vi "FGV_REF_EDITOR_records_display.vi"(4 "front_panel_reference":refnum<vi>, 6 "SQL_listbox_reference":refnum<vi>, 7 "options":T3, 8 "error_in":errorcluster, 10 "uneditable_columns":string[](array[string])=["ID", "CREATION_TIME", "CREATED_BY"], 11 "input":variant) -> (0 "error_out":errorcluster, 1 "all_info":T1, 2 "array_param_output":string[](array[string]), 3 "string_param_output":string)   [LabVIEW 2019]
uses:
  FGV_REF_EDITOR_records_display.ctl
  REF_EDITOR_all_info.ctl
  MAIN/SQL_record_states.ctl
  ini/typedef/CLIENT_all_config_info.ctl
  ini/typedef/CLIENT_main_ini_file.ctl
  queues/typedef/CLIENT_queue_refnums.ctl
  queues/typedef/SQL_EDITOR_queue_element.ctl
  MAIN/SQL_EDITOR/SQL_EDITOR_sequence_state.ctl
  queues/typedef/CLIENT_SCANNER_queue_element.ctl
  MAIN/SCANNER/SCANNER_sequence_state.ctl
  queues/typedef/CLIENT_REF_CHG_queue_element.ctl
  MAIN/reference_changed_connection/CLIENT_REF_CHG_sequence_state.ctl
  login/FGV_login.ctl
  <userlib>/_OpenG.lib/array/array.llb/Filter 1D Array (String)__ogtk.vi
  <userlib>/_OpenG.lib/array/array.llb/Delete Elements from 1D Array (I32)__ogtk.vi
  <vilib>/addons/database/_DB Variant To Data/Database Variant To Data.xnode
panel:
  out "data":string[][](array[string])
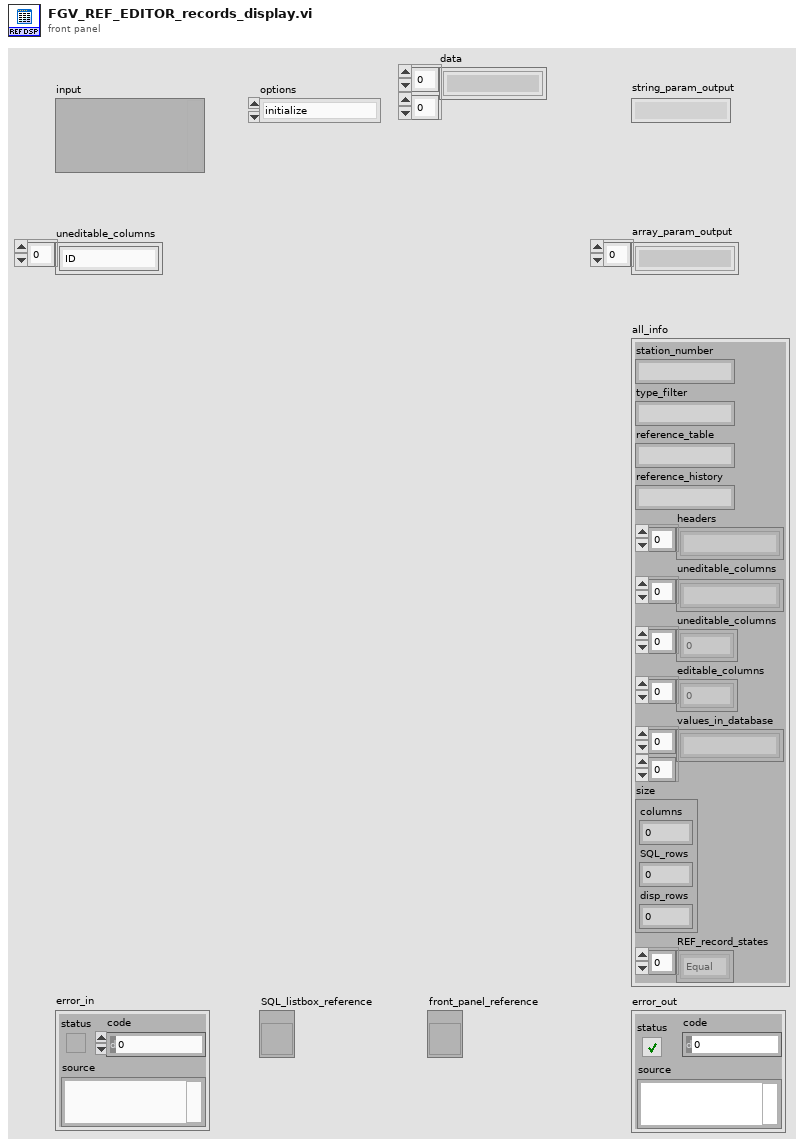
[diagram p1: front panel]
types:
  T1 = typedef "REF_EDITOR_all_info.ctl" = cluster{"station_number":string, "type_filter":string, "reference_table":string, "reference_history":string, "headers":string[], "uneditable_columns":string[], "uneditable_columns":i32[], "editable_columns":i32[], "values_in_database":string[][], "size":cluster{"columns":i32, "SQL_rows":i32, "disp_rows":i32}, "REF_record_states":T2[]}
  T2 = typedef "SQL_record_states.ctl" = enum16{"Equal", "Added", "Edited", "Deleted"}
  T3 = typedef "FGV_REF_EDITOR_records_display.ctl" = enum16{"initialize", "set_reference_tables_names", "set_station_number", "set_type_filter", "set_headers", "set_records", "get_ref_table_name", "get_ref_hist_table_name", "get_station_number", "get_type_filter", "get_headers", "get_uneditable_columns", "get_all_info", "record_added?", "record_inserted?", "record_edited?", "record_updated?", "record_deleted?", "discard_changes"}
  T4 = typedef "CLIENT_all_config_info.ctl" = cluster{"main_ini_file":T5, "SQL Password":string, "queue_refnums":T6}
  T5 = typedef "CLIENT_main_ini_file.ctl" = cluster{"SQL Driver":string, "SQL Server":string, "SQL Database":string, "SQL UID":string, "Reference table":string, "Reference history":string, "Archivisation CFG table":string, "Archivisation CFG history":string, "User table":string, "User history":string, "logout timeout [ms]":i32, "records per page":i32, "default language":string, "REF CHG connection IP":string, "REF CHG remote port":i32, "REF CHG local port":i32, "SCANNER COM port":u16, "SCANNER Baud rate":u32, "SCANNER Data bits":u16, "SCANNER Pairity":enum16{"None", "Odd", "Even", "Mark", "Space"}, "SCANNER Stop bits":u16, "SCANNER Flow control":u16, "SCANNER Termination char":u8}
  T6 = typedef "CLIENT_queue_refnums.ctl" = cluster{"SQL_EDITOR_queue":refnum<queue>, "SCANNER_queue":refnum<queue>, "SCANNER_data":refnum<queue>, "CLIENT_REF_CHG_queue":refnum<queue>}
  T7 = typedef "FGV_login.ctl" = enum16{"initialize", "login", "logout", "get_login_info"}
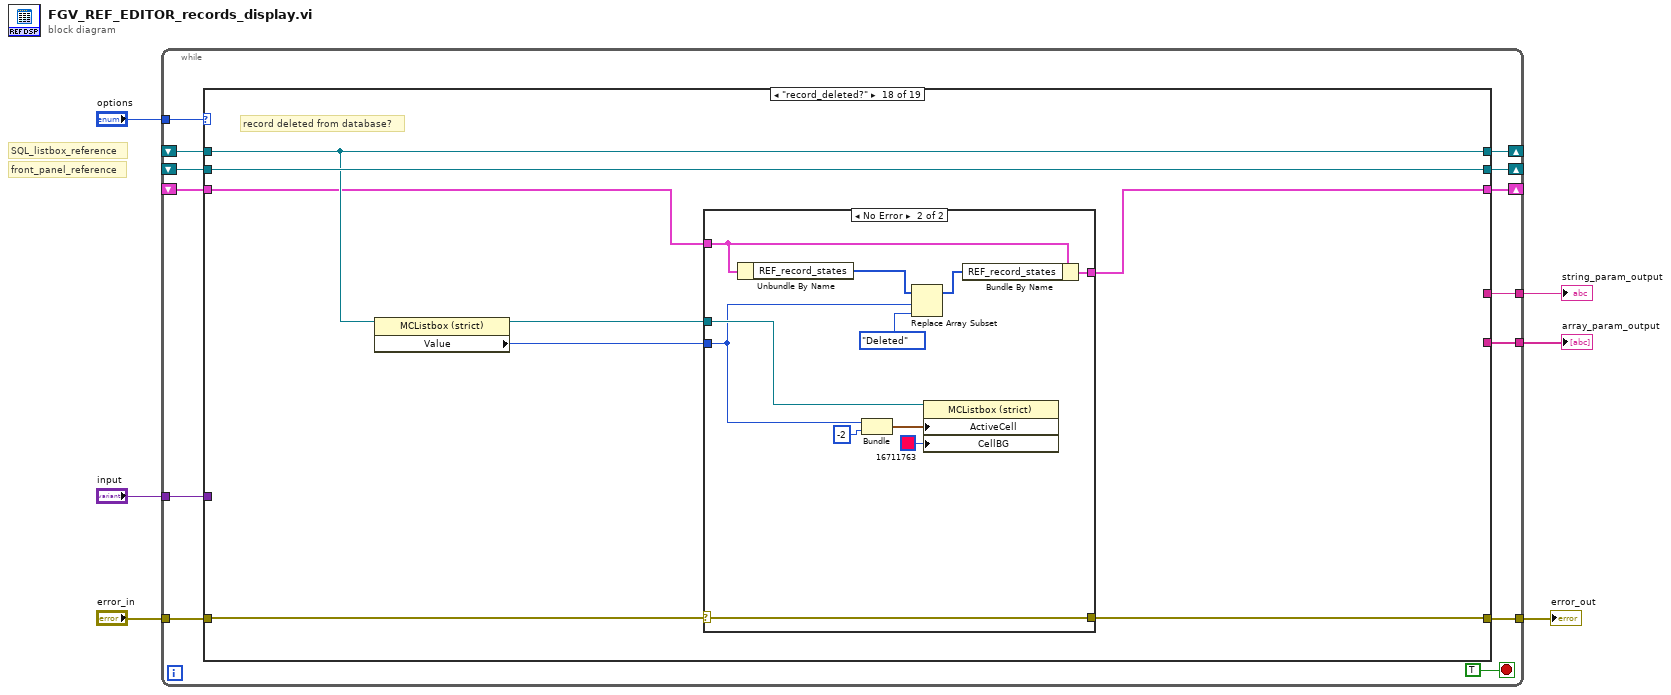
[diagram p0: block diagram]
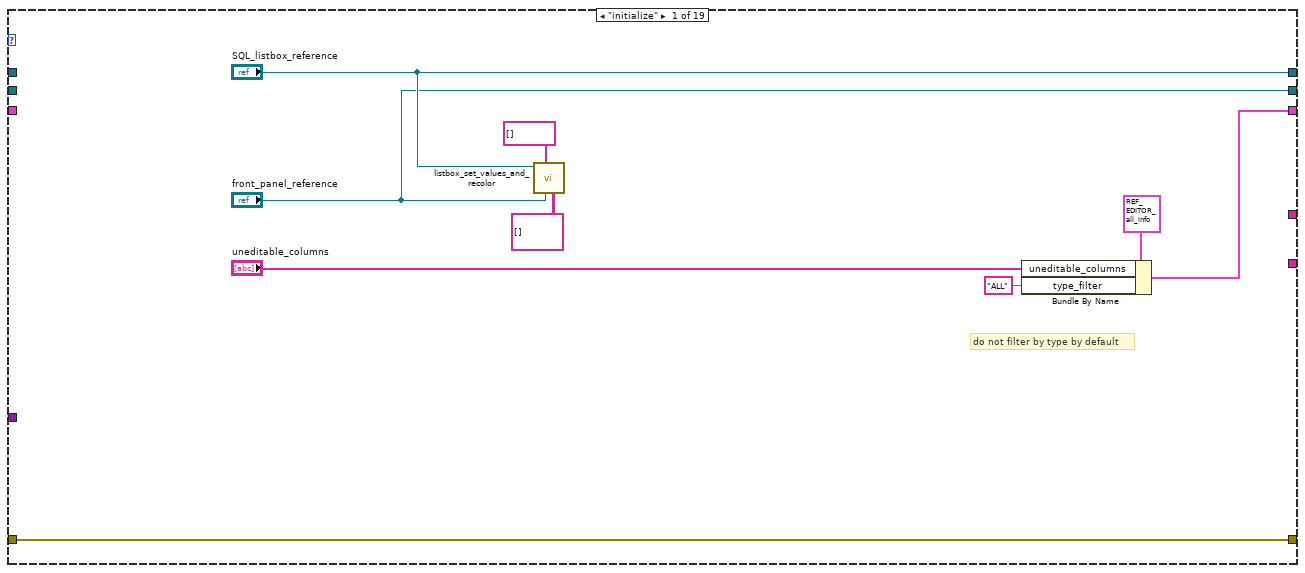
[diagram p2: hidden frame]
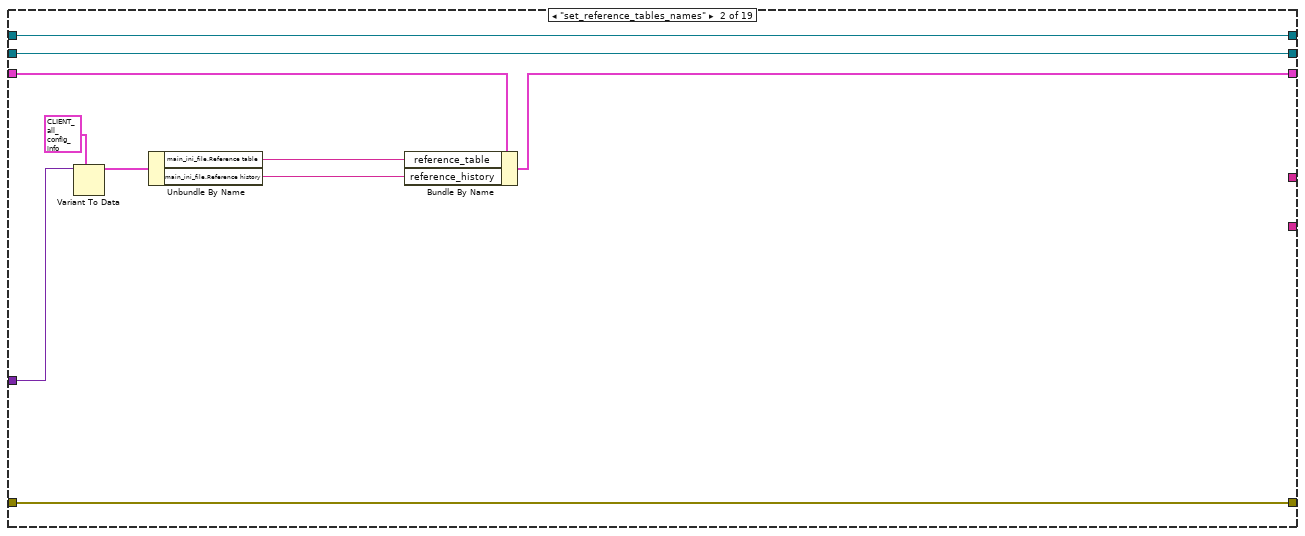
[diagram p3: hidden frame]
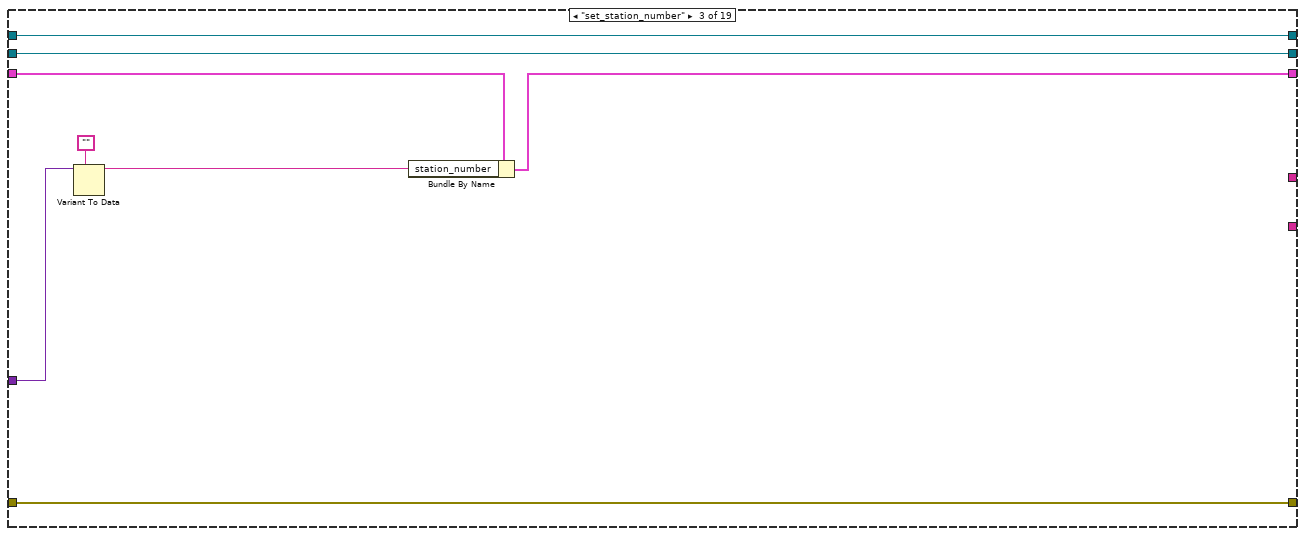
[diagram p4: hidden frame]
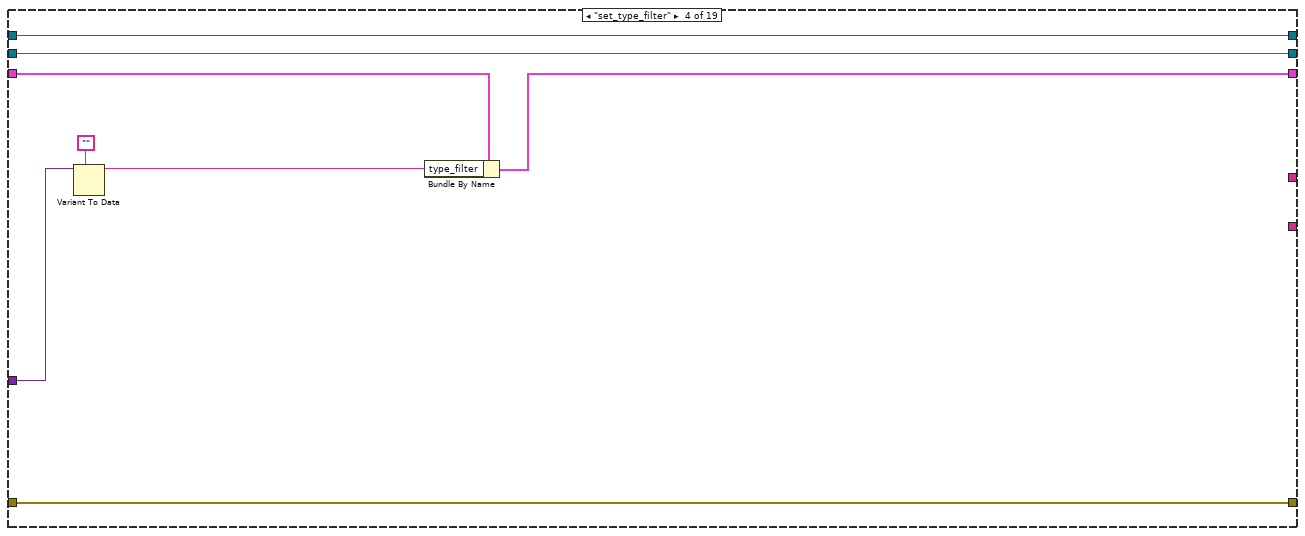
[diagram p5: hidden frame]
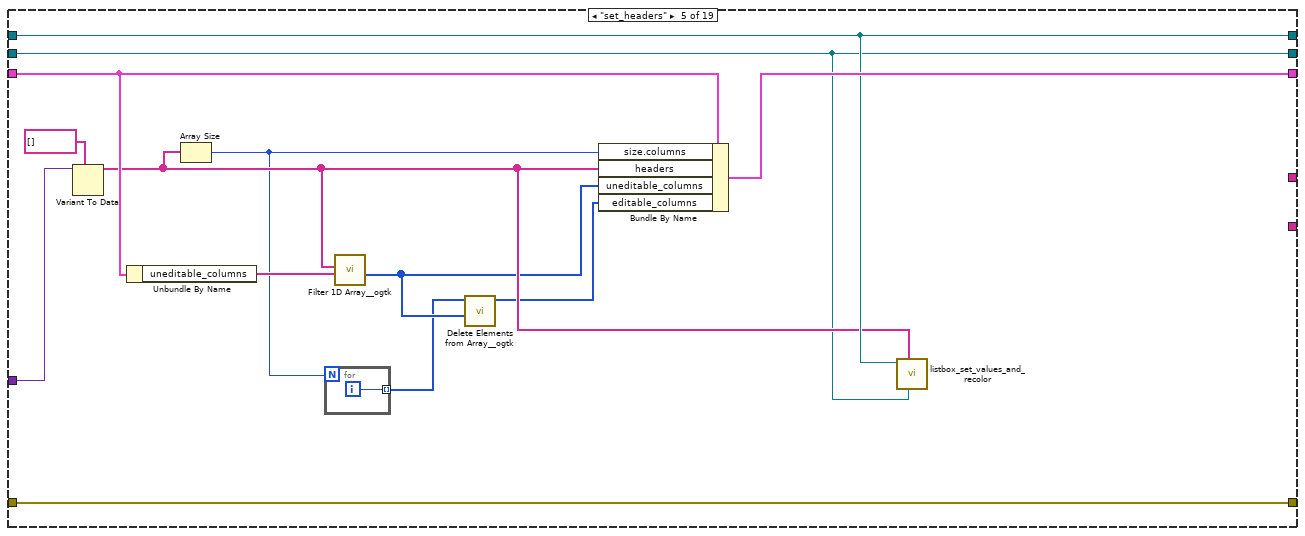
[diagram p6: hidden frame]
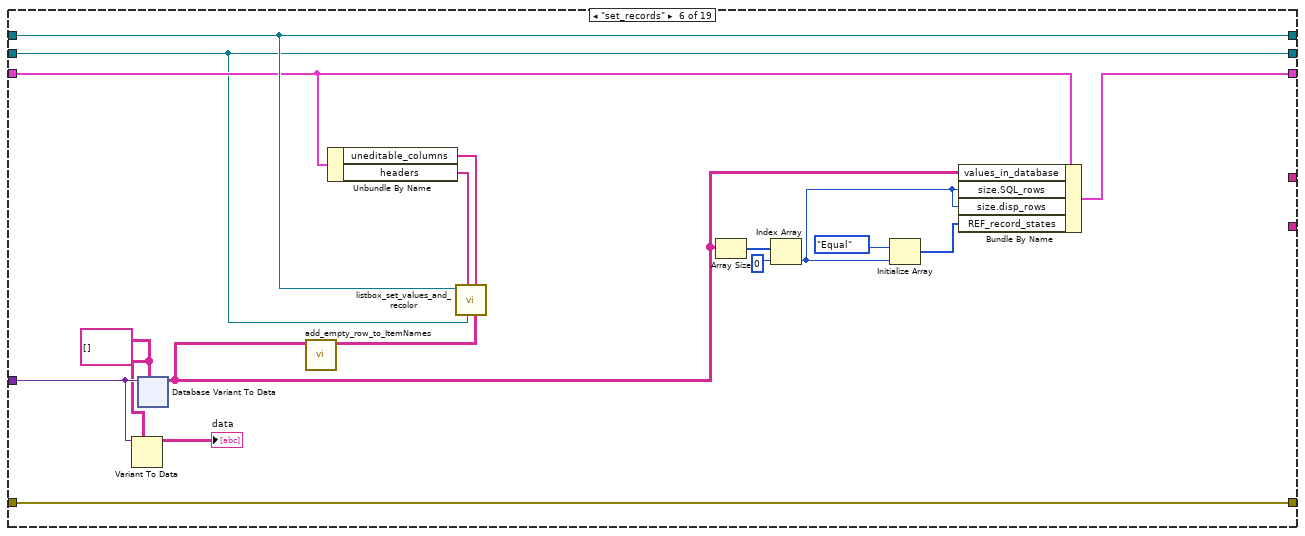
[diagram p7: hidden frame]
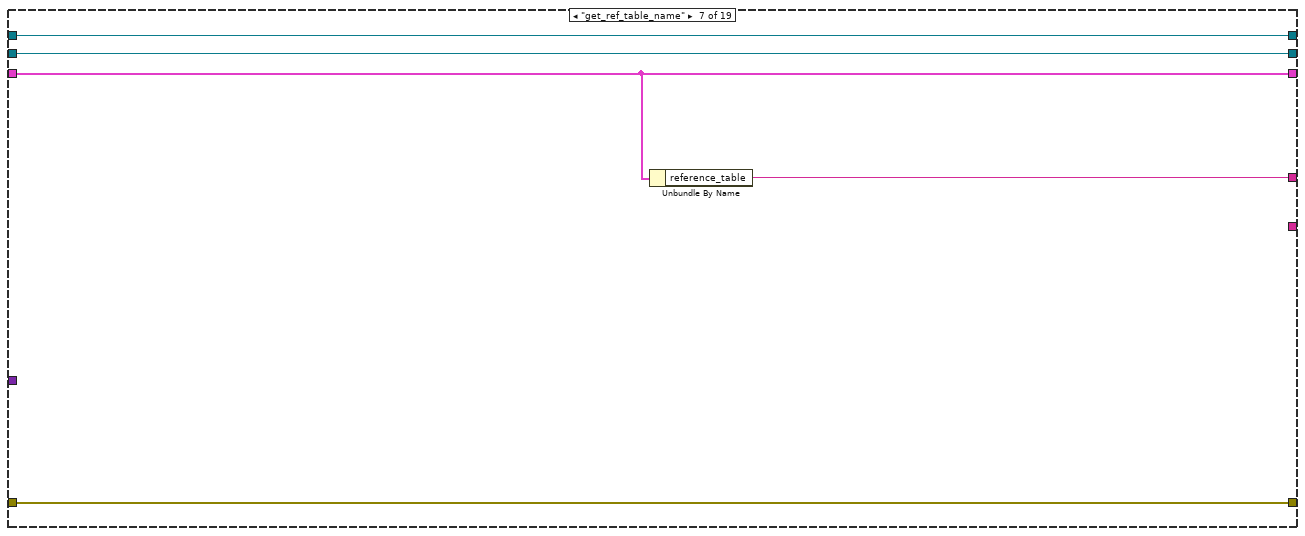
[diagram p8: hidden frame]
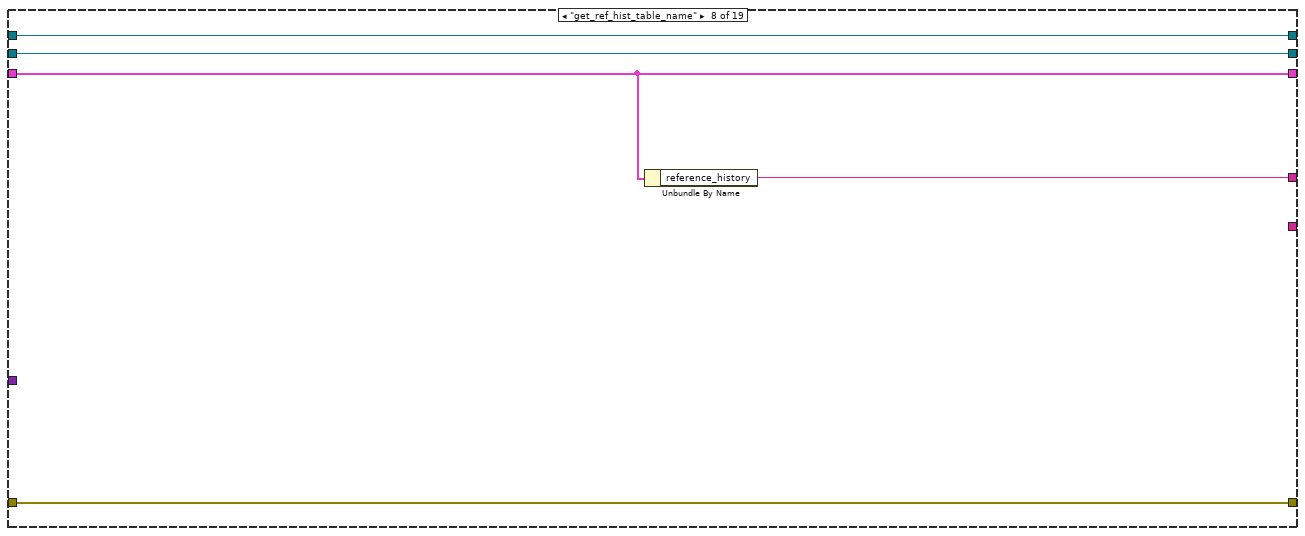
[diagram p9: hidden frame]
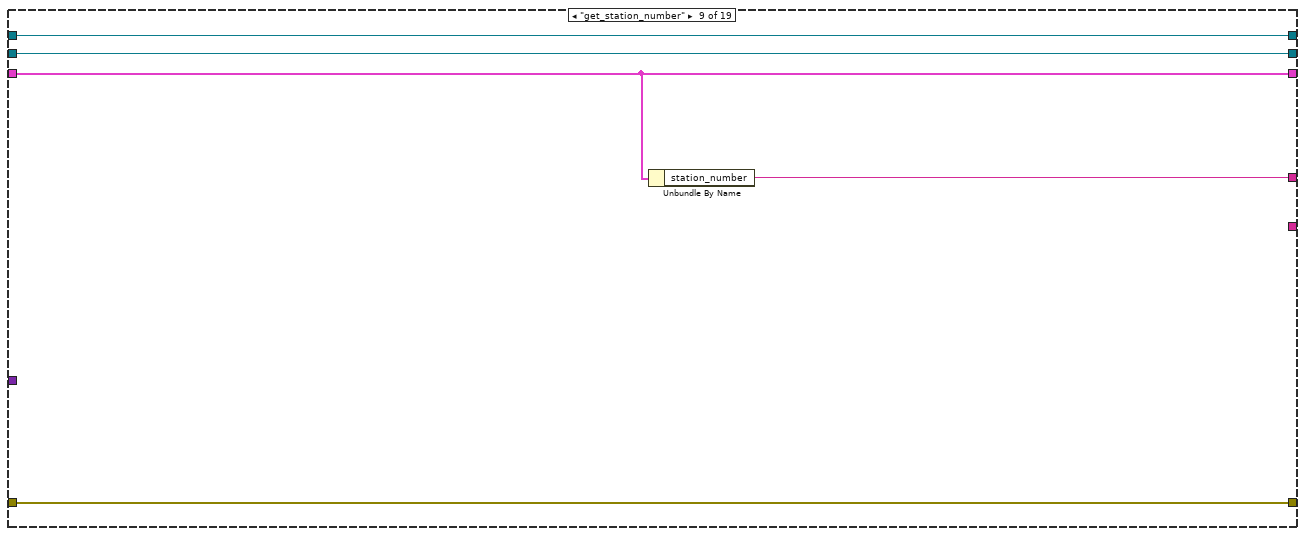
[diagram p10: hidden frame]
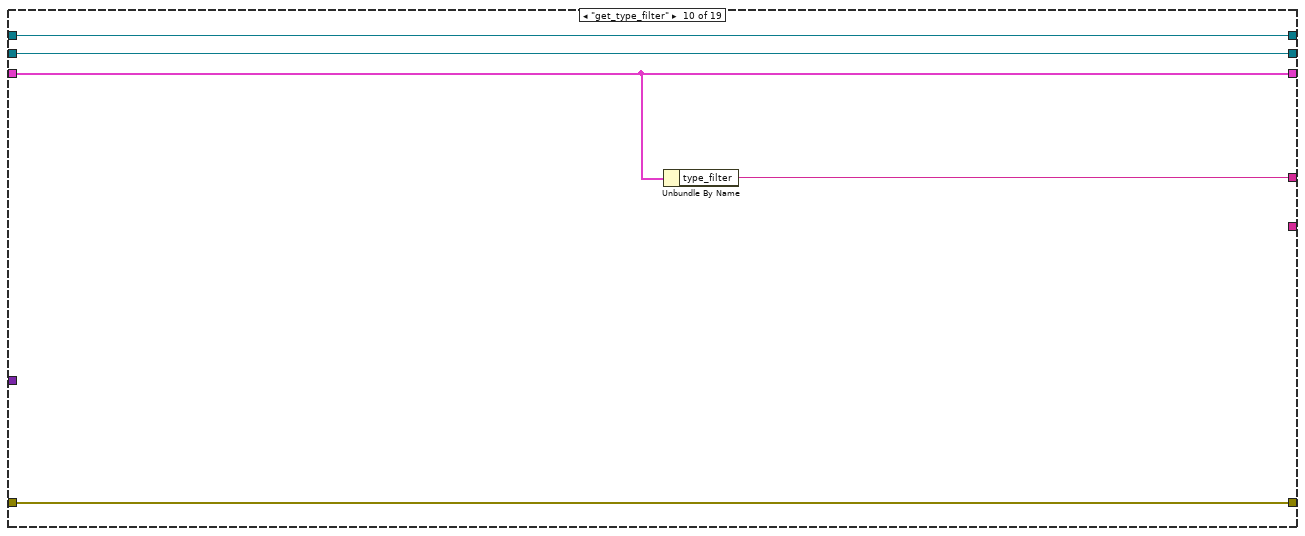
[diagram p11: hidden frame]
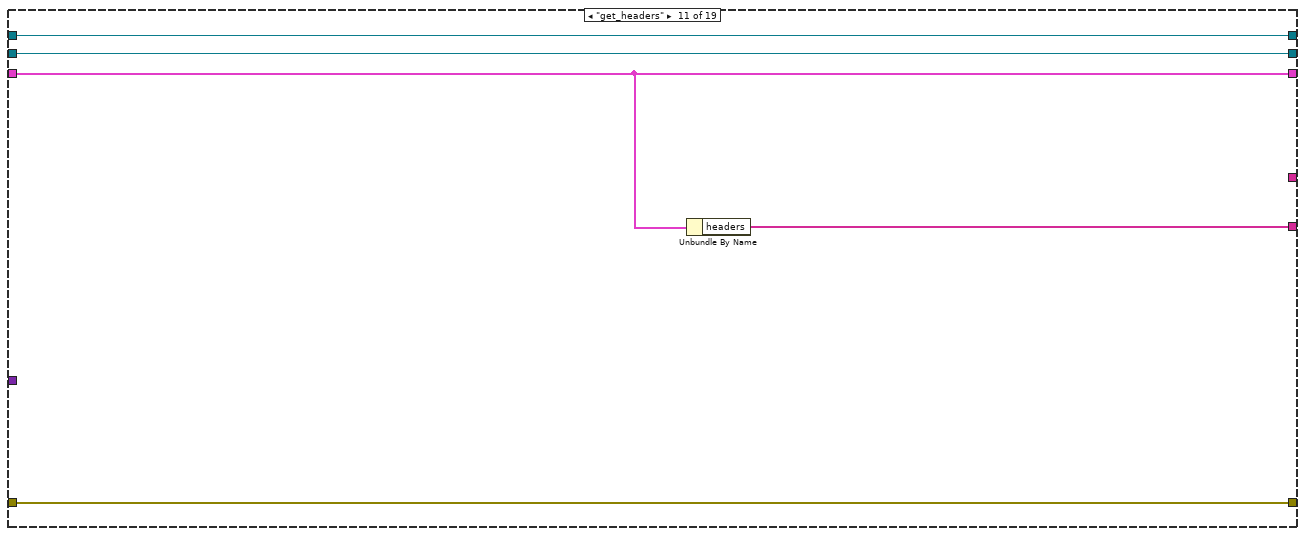
[diagram p12: hidden frame]
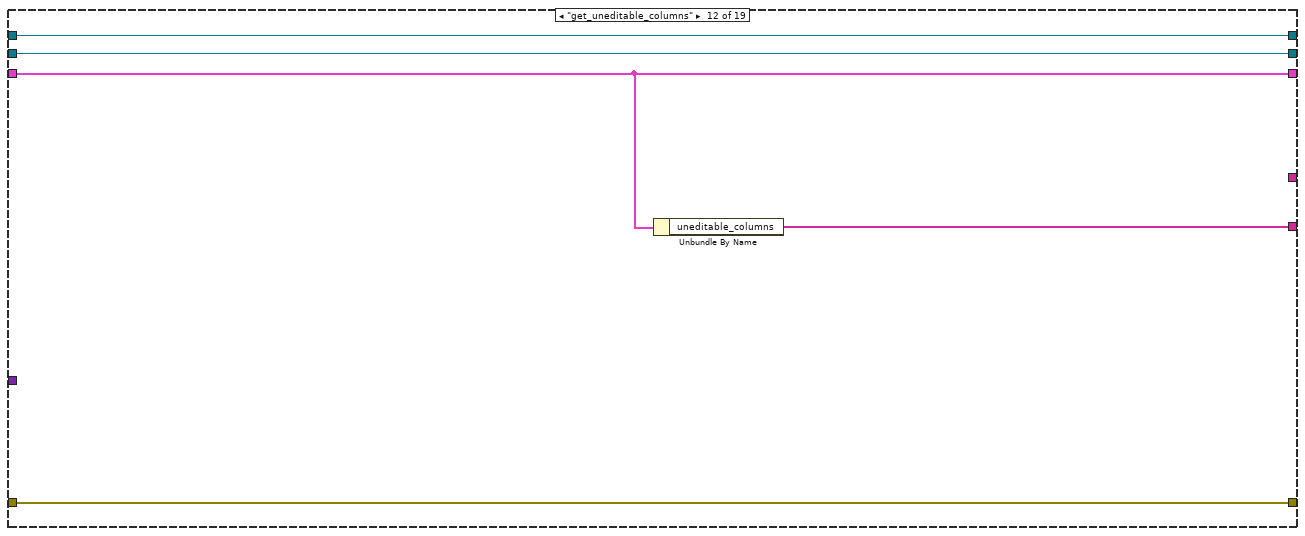
[diagram p13: hidden frame]
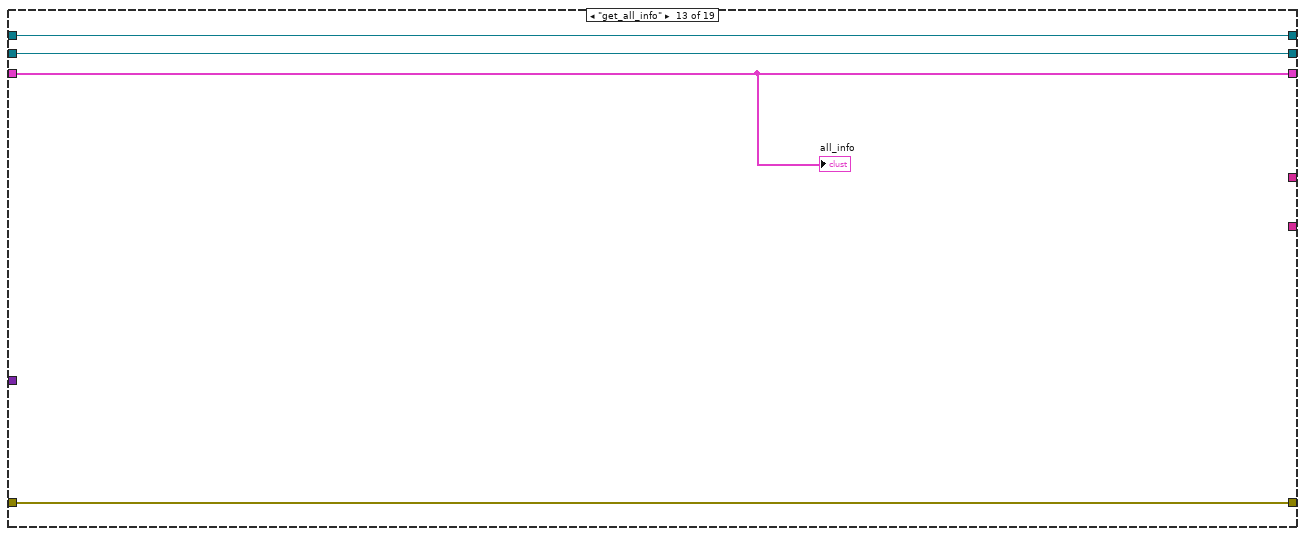
[diagram p14: hidden frame]
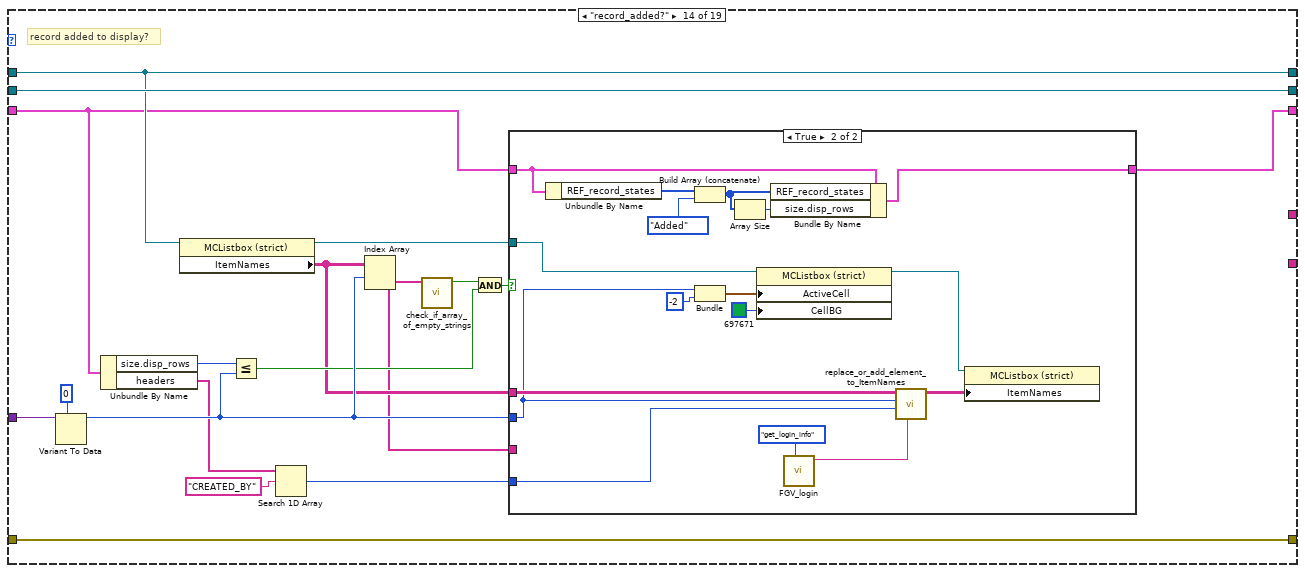
[diagram p15: hidden frame]
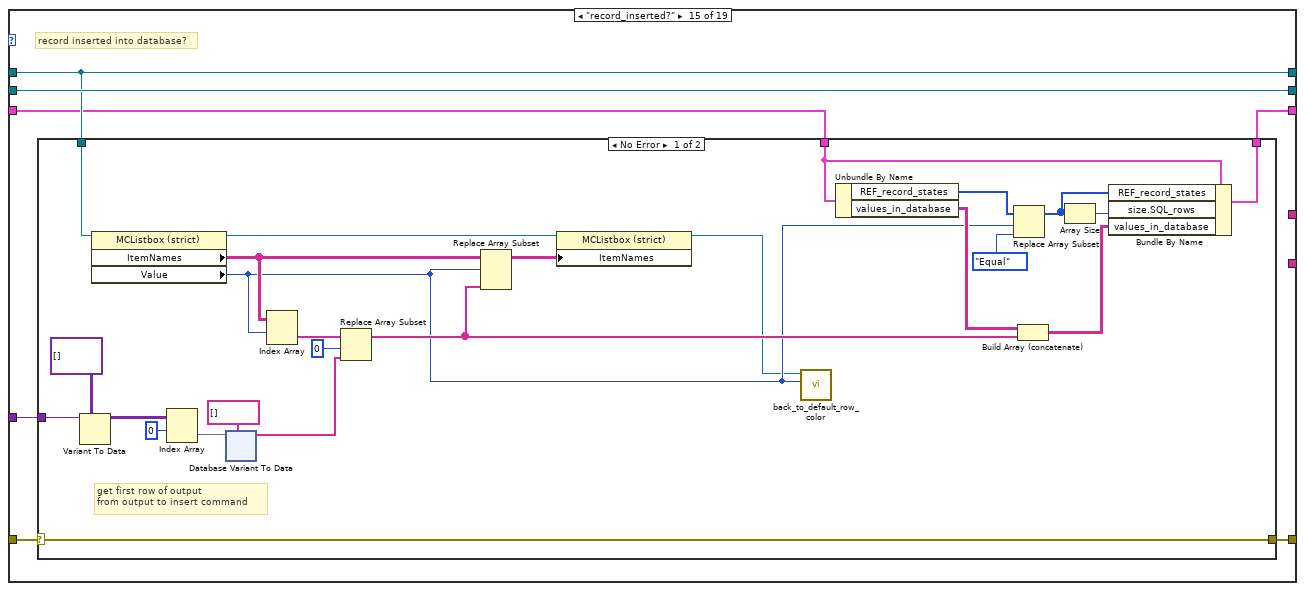
[diagram p17: hidden frame]
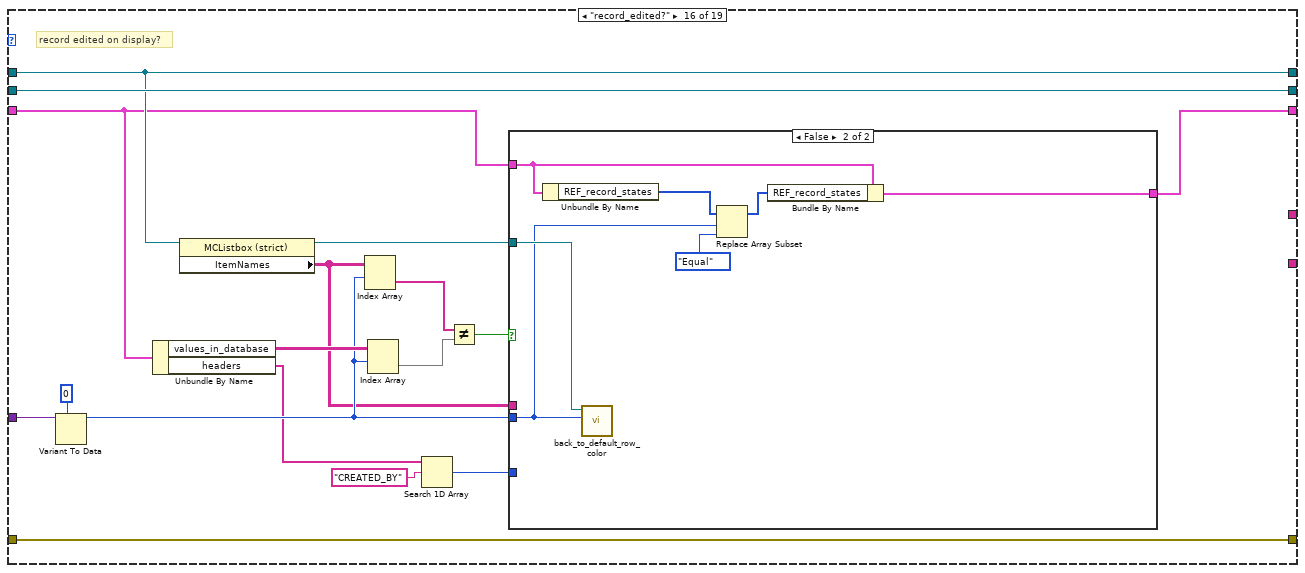
[diagram p19: hidden frame]
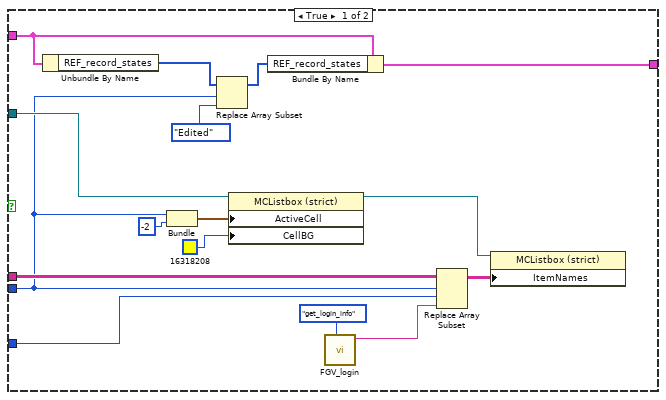
[diagram p20: hidden frame]
diagram:
  # "front_panel_reference"
  # "SQL_listbox_reference"
  n1 = while {
    tunnel: "options" -> [w18]
    tunnel: [w17] -> w6
    tunnel: "error_in" -> [w16]
    shift-right: [w15] -> _
    shift-left: _ -> [w14]
    tunnel: [w13] -> w3
    shift-right: [w12] -> _
    shift-left: _ -> [w11]
    tunnel: [w10] -> w2
    tunnel: "input" -> [w9]
    shift-right: [w8] -> _
    shift-left: _ -> [w7]
    stop <- TRUE stop-if-true
    n2 = case shown="\"record_deleted?\"" w18 {
      tunnel: [w28 w38 w46 w54 w67 w85 w120 w125 w130 w135 w141 w146 w150 w169 w189 w276 w305 w373 w398] -> w17
      tunnel: w16 -> [w28 w38 w46 w54 w67 w85 w120 w125 w130 w135 w141 w146 w150 w169 w193 w276 w304 w374 w398]
      tunnel: [w24 w36 w44 w52 w66 w81 w122 w127 w132 w137 w142 w147 w151 w163 w190 w264 w301 w375 w399] -> w15
      tunnel: w14 -> [_ w37 w45 w53 w62 w82 w122 w127 w132 w137 w142 w147 w151 w161 w191 w265 w302 w376 w394]
      tunnel: [_ _ _ _ _ _ w121 w126 w131 w136 _ _ _ _ _ _ _ _ _] -> w13
      tunnel: ["SQL_listbox_reference" w35 w43 w51 w63 w84 w119 w124 w129 w134 w138 w145 w149 w165 w192 w271 w303 w378 w393] -> w12
      tunnel: w11 -> [_ w35 w43 w51 w63 w84 w119 w124 w129 w134 w138 w145 w149 w165 w192 w271 w303 w378 w393]
      tunnel: [_ _ _ _ _ _ _ _ _ _ w140 w144 _ _ _ _ _ _ _] -> w10
      tunnel: w9 -> [_ w34 w42 w50 w65 w74 _ _ _ _ _ _ _ w167 w188 w274 w300 _ _]
      tunnel: ["front_panel_reference" w33 w39 w47 w55 w69 w118 w123 w128 w133 w139 w143 w148 w168 w194 w275 w306 w379 w401] -> w8
      tunnel: w7 -> [_ w33 w39 w47 w55 w69 w118 w123 w128 w133 w139 w143 w148 w168 w194 w275 w306 w379 w401]
      frame "initialize" {
        # "do not filter by type by default"
        n3 = call "listbox_set_values_and_recolor.vi"("item_names"=string[][] [], "front_panel_reference"="front_panel_reference", "column_names"=string[] [], "multicolumn_listbox_reference_in"="SQL_listbox_reference") -> ()  [unwired: 6 in, 2 out]
        n4 = Bundle By Name(cluster=T1 {"station_number"="", "type_filter"="", "reference_table"="", "reference_history"="", "headers"=[], "uneditable_columns"=[], "uneditable_columns"=[], "editable_columns"=[], "values_in_database"=[], "size"={"columns"=0, "SQL_rows"=0, "disp_rows"=0}, "REF_record_states"=[]} ("SQL_selection"), "uneditable_columns"="uneditable_columns", "type_filter"="ALL") -> (w24:T1)
      }
      frame "set_reference_tables_names" {
        n5 = Variant To Data(type=T4 {"main_ini_file"={"SQL Driver"="", "SQL Server"="", "SQL Database"="", "SQL UID"="", "Reference table"="", "Reference history"="", "Archivisation CFG table"="", "Archivisation CFG history"="", "User table"="", "User history"="", "logout timeout [ms]"=0, "records per page"=0, "default language"="", "REF CHG connection IP"="", "REF CHG remote port"=0, "REF CHG local port"=0, "SCANNER COM port"=0, "SCANNER Baud rate"=0, "SCANNER Data bits"=0, "SCANNER Pairity"=enum."None", "SCANNER Stop bits"=10, "SCANNER Flow control"=0, "SCANNER Termination char"=0}, "SQL Password"="", "queue_refnums"={"SQL_EDITOR_queue"=refnum, "SCANNER_queue"=refnum, "SCANNER_data"=refnum, "CLIENT_REF_CHG_queue"=refnum}} ("all_config_info_out"), Variant=w34) -> (data=w31:T4)  [unwired: 1 in, 1 out]
        n6 = Unbundle By Name(w31) -> ("main_ini_file.Reference table"=w30:string, "main_ini_file.Reference history"=w29:string)
        n7 = Bundle By Name(cluster=w37, "reference_table"=w30, "reference_history"=w29) -> (w36:T1)
      }
      frame "set_station_number" {
        n8 = Variant To Data(type="", Variant=w42) -> (data=w40:string)  [unwired: 1 in, 1 out]
        n9 = Bundle By Name(cluster=w45, "station_number"=w40) -> (w44:T1)
      }
      frame "set_type_filter" {
        n10 = Variant To Data(type="", Variant=w50) -> (data=w48:string)  [unwired: 1 in, 1 out]
        n11 = Bundle By Name(cluster=w53, "type_filter"=w48) -> (w52:T1)
      }
      frame "set_headers" {
        n12 = Variant To Data(type=string[] [], Variant=w65) -> (data=w61:string[])  [unwired: 1 in, 1 out]
        n13 = Unbundle By Name(w62) -> ("uneditable_columns"=w59:string[])
        n14 = Array Size(array=w61) -> (size(s)=w56:i32)
        n15 = for {
          N: w56 -> [_]
          tunnel: [w68] -> w58 mode=indexing
          i -> [w68]
        }
        n16 = call-poly <userlib>:"Filter 1D Array__ogtk.vi"("items to filter"=w59, "array"=w61) -> ("filtered item indices"=w60:i32[])  [unwired: 4 in, 1 out]
        n17 = call-poly <userlib>:"Delete Elements from Array__ogtk.vi"("indices"=w60, "array"=w58) -> ("array w/ subset deleted"=w57:i32[])  [unwired: 8 in, 1 out]
        n18 = Bundle By Name(cluster=w62, "size.columns"=w56, "headers"=w61, "uneditable_columns"=w60, "editable_columns"=w57) -> (w66:T1)
        n19 = call "listbox_set_values_and_recolor.vi"("front_panel_reference"=w55, "column_names"=w61, "multicolumn_listbox_reference_in"=w63) -> ()  [unwired: 7 in, 2 out]
      }
      frame "set_records" {
        w73 = string[][] []
        n20 = Variant To Data(type=w73, Variant=w74) -> (data=→"data":string[][])  [unwired: 1 in, 1 out]
        n21 = xnode "Database Variant To Data"("database variant"=w74, "type"=w73) -> ("data"=w71:string[][])  [unwired: 1 in, 1 out]
        n22 = call "add_empty_row_to_ItemNames.vi"("ItemNames_in"=w71) -> ("ItemNames_out"=w70:string[][])  [unwired: 10 in]
        n23 = Unbundle By Name(w82) -> ("uneditable_columns"=w75:string[], "headers"=w83:string[])
        n24 = call "listbox_set_values_and_recolor.vi"("item_names"=w70, "uneditable_columns"=w75, "front_panel_reference"=w69, "column_names"=w83, "multicolumn_listbox_reference_in"=w84) -> ()  [unwired: 5 in, 2 out]
        n25 = Array Size(array=w71) -> (size(s)=w80:i32[])
        n26 = Index Array(array=w80, index=0) -> (element=w77:i32)
        n27 = Initialize Array(SQL_record_states."Equal", w77) -> (w76:T2[])
        n28 = Bundle By Name(cluster=w82, "values_in_database"=w71, "size.SQL_rows"=w77, "size.disp_rows"=w77, "REF_record_states"=w76) -> (w81:T1)
      }
      frame "get_ref_table_name" {
        n29 = Unbundle By Name(w122) -> ("reference_table"=w121:string)
      }
      frame "get_ref_hist_table_name" {
        n30 = Unbundle By Name(w127) -> ("reference_history"=w126:string)
      }
      frame "get_station_number" {
        n31 = Unbundle By Name(w132) -> ("station_number"=w131:string)
      }
      frame "get_type_filter" {
        n32 = Unbundle By Name(w137) -> ("type_filter"=w136:string)
      }
      frame "get_headers" {
        n33 = Unbundle By Name(w142) -> ("headers"=w140:string[])
      }
      frame "get_uneditable_columns" {
        n34 = Unbundle By Name(w147) -> ("uneditable_columns"=w144:string[])
      }
      frame "get_all_info" {
        "all_info" <- w151
      }
      frame "record_added?" {
        # "record added to display?"
        n35 = Variant To Data(type=0, Variant=w167) -> (data=w159:i32)  [unwired: 1 in, 1 out]
        n36 = Unbundle By Name(w161) -> ("size.disp_rows"=w160:i32, "headers"=w154:string[])
        n37 = property class="MCListbox (strict)"(reference=w165) -> (reference out=w164:refnum<vi>, "ItemNames"=w156:string[][])  [unwired: 1 in, 1 out]
        n38 = Less Or Equal?(x=w160, y=w159) -> (x <= y?=w158:bool)
        n39 = Search 1D Array(1D array=w154, element="CREATED_BY") -> (index of element=w152:i32)  [unwired: 1 in]
        n40 = Index Array(array=w156, index (row)=w159) -> (element=w155:string[])  [unwired: 1 in]
        n41 = call "check_if_array_of_empty_strings.vi"("array"=w155) -> ("Not empty?"=w157:bool)  [unwired: 10 in]
        n42 = And(x=w157, y=w158) -> (x .and. y?=w162:bool)
        n43 = case shown="True" w162 {
          tunnel: w159 -> [_ w176]
          tunnel: w164 -> [_ w184]
          tunnel: w161 -> [w170 w182]
          tunnel: [w170 w183] -> w163
          tunnel: w156 -> [_ w177]
          tunnel: w155 -> [_ _]
          tunnel: w152 -> [_ w175]
          frame False {
          }
          frame True {
            n44 = Unbundle By Name(w182) -> ("REF_record_states"=w181:T2[])
            n45 = Build Array (concatenate)(w181, SQL_record_states."Added" ("new element/subarray")) -> (w179:T2[])
            n46 = Bundle(w176, -2) -> (w185:cluster{i32, i32})  [unwired: 1 in]
            n47 = Array Size(array=w179) -> (size(s)=w178:i32)
            n48 = property on="Property Node" class="MCListbox (strict)"(reference=w184, "ActiveCell"=w185, "CellBG"=u32 697671) -> (reference out=w172:refnum<vi>)  [unwired: 1 in, 1 out]
            n49 = Bundle By Name(cluster=w182, "REF_record_states"=w179, "size.disp_rows"=w178) -> (w183:T1)
            n50 = call "FGV_login.vi"("options"=FGV_login."get_login_info") -> ("username_out"=w173:string)  [unwired: 8 in, 2 out]
            n51 = call "replace_or_add_element_to_ItemNames.vi"("element"=w173, "column"=w175, "row"=w176, "ItemNames_in"=w177) -> ("ItemNames_out"=w171:string[][])  [unwired: 7 in]
            n52 = property class="MCListbox (strict)"(reference=w172, "ItemNames"=w171) -> ()  [unwired: 1 in, 2 out]
          }
        }
      }
      frame "record_inserted?" {
        # "record inserted into database?"
        n53 = case shown="No Error" w193 {
          selector: w193 -> [w198 w259]
          tunnel: w191 -> [w219 w258]
          tunnel: [w218 w258] -> w190
          tunnel: w188 -> [w203 _]
          tunnel: w192 -> [w202 _]
          tunnel: [w198 w259] -> w189
          frame No Error {
            # "get first row of output\nfrom output to insert command"
            n54 = Variant To Data(type=variant[][] [], Variant=w203) -> (data=w210:variant[][])  [unwired: 1 in, 1 out]
            n55 = property class="MCListbox (strict)"(reference=w202) -> (reference out=w197:refnum<vi>, "ItemNames"=w204:string[][], "Value"=w200:i32)  [unwired: 1 in, 1 out]
            n56 = Index Array(array=w210, index (row)=0) -> (element=w207:variant[])  [unwired: 1 in]
            n57 = xnode "Database Variant To Data"("database variant"=w207, "type"=string[] []) -> ("data"=w205:string[])  [unwired: 1 in, 1 out]
            n58 = Index Array(array=w204, index (row)=w200) -> (element=w209:string[])  [unwired: 1 in]
            n59 = Replace Array Subset(array=w209, new element=w205, index=0) -> (w201:string[])
            n60 = Replace Array Subset(array=w204, new element=w201, index (row)=w200) -> (w195:string[][])  [unwired: 1 in]
            n61 = property class="MCListbox (strict)"(reference=w197, "ItemNames"=w195) -> (reference out=w196:refnum<vi>)  [unwired: 1 in, 1 out]
            n62 = call "back_to_default_row_color.vi"("row"=w200, "listbox_reference"=w196) -> ()  [unwired: 9 in, 1 out]
            n63 = Unbundle By Name(w219) -> ("REF_record_states"=w216:T2[], "values_in_database"=w215:string[][])
            n64 = Replace Array Subset(array=w216, new element=SQL_record_states."Equal" ("new element/subarray"), index=w200) -> (w212:T2[])
            n65 = Build Array (concatenate)(w215, w201) -> (w214:string[][])
            n66 = Array Size(array=w212) -> (size(s)=w213:i32)
            n67 = Bundle By Name(cluster=w219, "REF_record_states"=w212, "size.SQL_rows"=w213, "values_in_database"=w214) -> (w218:T1)
          }
          frame Error {
          }
        }
      }
      frame "record_edited?" {
        # "record edited on display?"
        n68 = Variant To Data(type=0, Variant=w274) -> (data=w266:i32)  [unwired: 1 in, 1 out]
        n69 = Unbundle By Name(w265) -> ("values_in_database"=w272:string[][], "headers"=w261:string[])
        n70 = property class="MCListbox (strict)"(reference=w271) -> (reference out=w267:refnum<vi>, "ItemNames"=w263:string[][])  [unwired: 1 in, 1 out]
        n71 = Index Array(array=w263, index (row)=w266) -> (element=w270:string[])  [unwired: 1 in]
        n72 = Index Array(array=w272, index (row)=w266) -> (element=w269:string[])  [unwired: 1 in]
        n73 = Search 1D Array(1D array=w261, element="CREATED_BY") -> (index of element=w260:i32)  [unwired: 1 in]
        n74 = Not Equal?(x=w270, y=w269) -> (x != y?=w268:bool)
        n75 = case shown="False" w268 {
          tunnel: w266 -> [w280 w293]
          tunnel: w267 -> [w290 w294]
          tunnel: w265 -> [w286 w297]
          tunnel: [w284 w295] -> w264
          tunnel: w263 -> [w281 _]
          tunnel: w260 -> [w279 _]
          frame True {
            n76 = Unbundle By Name(w286) -> ("REF_record_states"=w287:T2[])
            n77 = Bundle(w280, -2) -> (w291:cluster{i32, i32})  [unwired: 1 in]
            n78 = Replace Array Subset(array=w287, new element=SQL_record_states."Edited" ("new element/subarray"), index=w280) -> (w285:T2[])
            n79 = property on="Property Node" class="MCListbox (strict)"(reference=w290, "ActiveCell"=w291, "CellBG"=u32 16318208) -> (reference out=w277:refnum<vi>)  [unwired: 1 in, 1 out]
            n80 = Bundle By Name(cluster=w286, "REF_record_states"=w285) -> (w284:T1)
            n81 = call "FGV_login.vi"("options"=FGV_login."get_login_info") -> ("username_out"=w282:string)  [unwired: 8 in, 2 out]
            n82 = Replace Array Subset(array=w281, new element=w282, index (row)=w280, index (col)=w279) -> (w278:string[][])
            n83 = property class="MCListbox (strict)"(reference=w277, "ItemNames"=w278) -> ()  [unwired: 1 in, 2 out]
          }
          frame False {
            n84 = Unbundle By Name(w297) -> ("REF_record_states"=w298:T2[])
            n85 = call "back_to_default_row_color.vi"("row"=w293, "listbox_reference"=w294) -> ()  [unwired: 9 in, 1 out]
            n86 = Replace Array Subset(array=w298, new element=SQL_record_states."Equal" ("new element/subarray"), index=w293) -> (w296:T2[])
            n87 = Bundle By Name(cluster=w297, "REF_record_states"=w296) -> (w295:T1)
          }
        }
      }
      frame "record_updated?" {
        # "record updated in database?"
        n88 = case shown="No Error" w304 {
          selector: w304 -> [w310 w370]
          tunnel: w303 -> [w331 _]
          tunnel: w302 -> [w330 w371]
          tunnel: [w329 w371] -> w301
          tunnel: w300 -> [w328 _]
          tunnel: [w310 w370] -> w305
          frame No Error {
            # "get first row of output\nfrom output to third command in ref update transaction"
            n89 = Variant To Data(type=variant[][][] [], Variant=w328) -> (data=w326:variant[][][])  [unwired: 1 in, 1 out]
            n90 = property class="MCListbox (strict)"(reference=w331) -> (reference out=w309:refnum<vi>, "ItemNames"=w318:string[][], "Value"=w317:i32)  [unwired: 1 in, 1 out]
            n91 = Index Array(array=w326, index (dim 0)=2 ("index (page)"), index (dim 1)=0 ("disabled index (row)")) -> (element=w321:variant[])  [unwired: 1 in]
            n92 = xnode "Database Variant To Data"("database variant"=w321, "type"=string[] []) -> ("data"=w319:string[])  [unwired: 1 in, 1 out]
            n93 = Index Array(array=w318, index (row)=w317) -> (element=w323:string[])  [unwired: 1 in]
            n94 = Replace Array Subset(array=w323, new element=w319, index=0) -> (w316:string[])
            n95 = Replace Array Subset(array=w318, new element=w316, index (row)=w317) -> (w307:string[][])  [unwired: 1 in]
            n96 = property class="MCListbox (strict)"(reference=w309, "ItemNames"=w307) -> (reference out=w308:refnum<vi>)  [unwired: 1 in, 1 out]
            n97 = Unbundle By Name(w330) -> ("REF_record_states"=w314:T2[], "values_in_database"=w311:string[][])
            n98 = call "back_to_default_row_color.vi"("row"=w317, "listbox_reference"=w308) -> ()  [unwired: 9 in, 1 out]
            n99 = Replace Array Subset(array=w311, new element=w316, index (row)=w317) -> (w312:string[][])  [unwired: 1 in]
            n100 = Replace Array Subset(array=w314, new element=SQL_record_states."Equal" ("new element/subarray"), index=w317) -> (w313:T2[])
            n101 = Bundle By Name(cluster=w330, "REF_record_states"=w313, "values_in_database"=w312) -> (w329:T1)
          }
          frame Error {
          }
        }
      }
      frame "record_deleted?" {
        # "record deleted from database?"
        n102 = property class="MCListbox (strict)"(reference=w378) -> (reference out=w377:refnum<vi>, "Value"=w372:i32)  [unwired: 1 in, 1 out]
        n103 = case shown="No Error" w374 {
          selector: w374 -> [w381 w382]
          tunnel: w377 -> [_ w390]
          tunnel: w376 -> [w380 w386]
          tunnel: [w380 w384] -> w375
          tunnel: [w381 w382] -> w373
          tunnel: w372 -> [_ w383]
          frame Error {
          }
          frame No Error {
            n104 = Unbundle By Name(w386) -> ("REF_record_states"=w387:T2[])
            n105 = Bundle("Value"=w383, -2) -> (w391:cluster{"Value":i32, i32})  [unwired: 1 in]
            n106 = Replace Array Subset(array=w387, new element=SQL_record_states."Deleted" ("new element/subarray"), index=w383) -> (w385:T2[])
            n107 = property on="Property Node" class="MCListbox (strict)"(reference=w390, "ActiveCell"=w391, "CellBG"=u32 16711763) -> ()  [unwired: 1 in, 2 out]
            n108 = Bundle By Name(cluster=w386, "REF_record_states"=w385) -> (w384:T1)
          }
        }
      }
      frame "discard_changes" {
        # "discard changes on display"
        n109 = property class="MCListbox (strict)"(reference=w393) -> (reference out=w400:refnum<vi>, "Value"=w396:i32)  [unwired: 1 in, 1 out]
        n110 = Unbundle By Name(w394) -> ("REF_record_states"=w397:T2[])
        n111 = Index Array(array=w397, index=w396) -> (element=w395:T2)
        n112 = case shown="\"Added\"" w395 {
          tunnel: w400 -> [_ w416 w422]
          tunnel: w394 -> [w402 w415 w431]
          tunnel: [w402 w414 w430] -> w399
          tunnel: w396 -> [_ w406 w421]
          tunnel: w394 -> [_ w411 w429]
          tunnel: w393 -> [_ w409 w427]
          frame Default {
          }
          frame "Edited" {
            n113 = Unbundle By Name(w411) -> ("values_in_database"=w407:string[][], "REF_record_states"=w410:T2[])
            n114 = property class="MCListbox (strict)"(reference=w409) -> (reference out=w403:refnum<vi>, "ItemNames"=w408:string[][])  [unwired: 1 in, 1 out]
            n115 = call "back_to_default_row_color.vi"("row"=w406, "listbox_reference"=w416) -> ()  [unwired: 9 in, 1 out]
            n116 = Index Array(array=w407, index (row)=w406) -> (element=w405:string[])  [unwired: 1 in]
            n117 = Replace Array Subset(array=w410, new element=SQL_record_states."Equal" ("new element/subarray"), index=w406) -> (w412:T2[])
            n118 = Replace Array Subset(array=w408, new element=w405, index (row)=w406) -> (w404:string[][])  [unwired: 1 in]
            n119 = property class="MCListbox (strict)"(reference=w403, "ItemNames"=w404) -> ()  [unwired: 1 in, 2 out]
            n120 = Bundle By Name(cluster=w415, "REF_record_states"=w412) -> (w414:T1)
          }
          frame "Added" {
            n121 = property class="MCListbox (strict)"(reference=w427) -> (reference out=w417:refnum<vi>, "ItemNames"=w426:string[][])  [unwired: 1 in, 1 out]
            n122 = Unbundle By Name(w429) -> ("REF_record_states"=w428:T2[])
            n123 = Bundle("Value"=w421, -2) -> (w425:cluster{"Value":i32, i32})  [unwired: 1 in]
            n124 = property on="Property Node" class="MCListbox (strict)"(reference=w422, "ActiveCell"=w425, "CellBG"=u32 16448250) -> ()  [unwired: 1 in, 2 out]
            n125 = Delete From Array(array=w428, index=w421) -> (array with subset deleted=w419:T2[])  [unwired: 1 in, 1 out]
            n126 = Delete From Array(array=w426, index (row)=w421) -> (array with subset deleted=w418:string[][])  [unwired: 2 in, 1 out]
            n127 = Array Size(array=w419) -> (size(s)=w420:i32)
            n128 = call "add_empty_row_to_ItemNames.vi"("multicolumn_listbox_reference_in"=w417, "ItemNames_in"=w418) -> ()  [unwired: 9 in, 1 out]
            n129 = Bundle By Name(cluster=w431, "size.disp_rows"=w420, "REF_record_states"=w419) -> (w430:T1)
          }
        }
      }
    }
  }
  "error_out" <- w6
  "string_param_output" <- w3
  "array_param_output" <- w2
